vi "ErrCheck_ZStackArray Present.vi"(8 "Error In":errorcluster, 11 "Settings ArrayIN":T1[](array[typedef])) -> (0 "Error Out":errorcluster, 2 "Error/Warning Message":string, 3 "Z-Stack data missing?":bool)   [LabVIEW 2012]
doc: "SciScan 1.2 160622"
uses:
  MacroGUI Module/Custom Controls and Typedefs/GFG Variable for IO.ctl
  GFG/GFG library.lvlib
  GFG/GFGnumericGet.vi
  GFG/GFGbooleanGet.vi
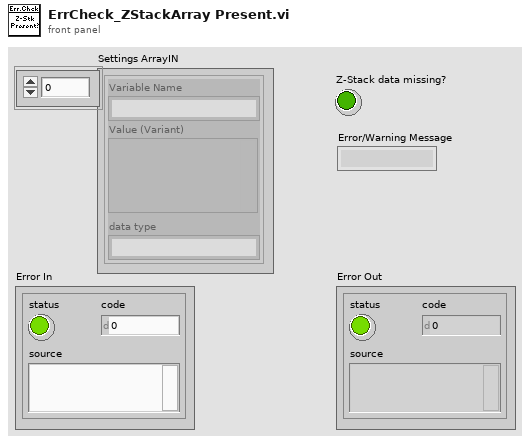
[diagram p1: front panel]
types:
  T1 = typedef "GFG Variable for IO.ctl" = cluster{"Variable Name":string, "Value (Variant)":variant, "data type":string}
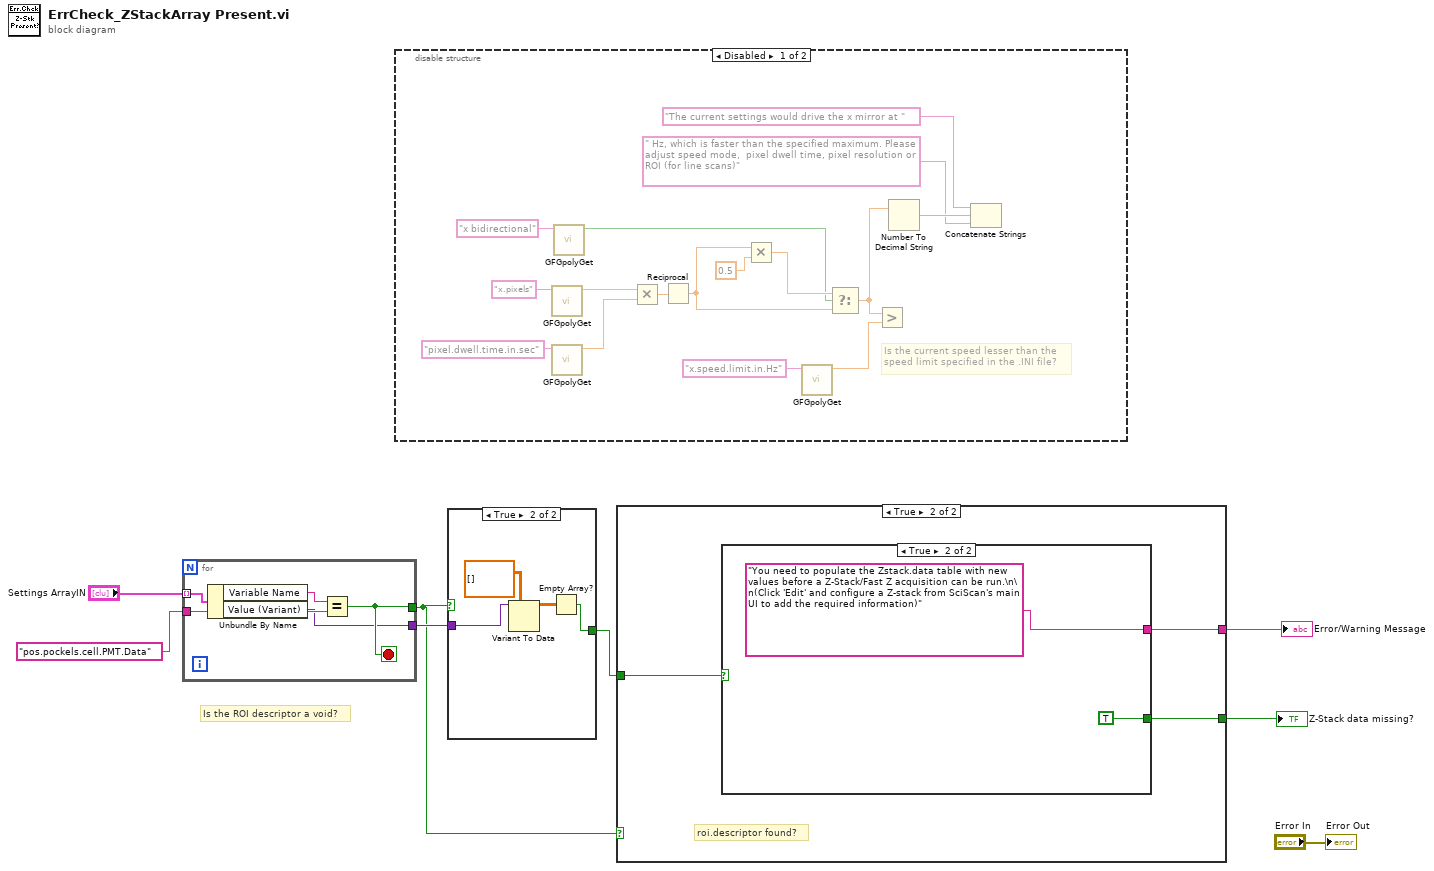
[diagram p0: block diagram]
diagram:
  # "Is the ROI descriptor a void?"
  n1 = for {
    tunnel: "Settings ArrayIN" -> [w13] mode=indexing
    tunnel: "pos.pockels.cell.PMT.Data" ("Variable Name in") -> [w11]
    tunnel: [w10] -> w2
    tunnel: [w9] -> w3
    stop <- w10 stop-if-true
    n2 = Unbundle By Name(w13) -> ("Variable Name"=w12:string, "Value (Variant)"=w9:variant)
    n3 = Equal?(x=w12, y=w11) -> (x = y?=w10:bool)
  }
  n4 = disable-structure shown="Disabled" {
    frame Disabled {
      # "Is the current speed lesser than the\nspeed limit specified in the .INI file?"
      n5 = call-poly "GFGpolyGet.vi"("Variable Name in"="x.pixels") -> ("Numeric"=w19:dbl)  [unwired: 8 in, 2 out]
      n6 = call-poly "GFGpolyGet.vi"("Variable Name in"="pixel.dwell.time.in.sec") -> ("Numeric"=w18:dbl)  [unwired: 8 in, 2 out]
      n7 = call-poly "GFGpolyGet.vi"("Variable Name in"="x bidirectional") -> ("Boolean Value OUT"=w20:bool)  [unwired: 9 in, 1 out]
      n8 = Multiply(x=w19, y=w18) -> (x*y=w21:dbl)
      n9 = Reciprocal(x=w21) -> (1/x=w22:dbl)
      n10 = Multiply(x=w22, y=0.5) -> (x*y=w23:dbl)
      n11 = call-poly "GFGpolyGet.vi"("Variable Name in"="x.speed.limit.in.Hz") -> ("Numeric"=w26:dbl)  [unwired: 8 in, 2 out]
      n12 = Select(t=w23, s=w20, f=w22) -> (s? t:f=w14:dbl)
      n13 = Greater?(x=w14, y=w26) -> ()  [unwired: 1 out]
      n14 = Number To Decimal String(number=w14) -> (decimal integer string=w16:string)  [unwired: 1 in]
      n15 = Concatenate Strings("The current settings would drive the x mirror at " ("message"), w16, " Hz, which is faster than the specified maximum. Please adjust speed mode,  pixel dwell time, pixel resolution or ROI (for line scans)" ("string")) -> ()  [unwired: 1 out]
    }
    frame Enabled {
    }
  }
  n16 = case shown="True" w2 {
    tunnel: w3 -> [_ w33]
    tunnel: [_ w31] -> w1
    frame False {
    }
    frame True {
      n17 = Variant To Data(type=dbl[][] [], Variant=w33) -> (data=w30:dbl[][])  [unwired: 1 in, 1 out]
      n18 = Empty Array?(array=w30) -> (empty?=w31:bool)
    }
  }
  n19 = case shown="True" w2 {
    tunnel: [_ w35] -> w7
    tunnel: w1 -> [_ w36]
    tunnel: [_ w34] -> w6
    frame False {
      # "Donot run the speed check for RESO system"
    }
    frame True {
      # "roi.descriptor found?"
      n20 = case shown="True" w36 {
        tunnel: [_ TRUE] -> w35
        tunnel: [_ "You need to populate the Zstack.data table with new values before a Z-Stack/Fast Z acquisition can be run.\n\n(Click 'Edit' and configure a Z-stack from SciScan's main UI to add the required information)" ("string")] -> w34
        frame False {
        }
        frame True {
        }
      }
    }
  }
  "Z-Stack data missing?" <- w7
  "Error/Warning Message" <- w6
  "Error Out" <- "Error In"
